vi "Variant to Byte Array.vi"(7 "InStruct":bool=TRUE, 8 "Error In":errorcluster, 10 "Byte Stream In":u8[](array[numeric]), 11 "Variant":variant) -> (0 "Error Out":errorcluster, 2 "Byte Stream Out":u8[](array[numeric]))   [LabVIEW 2020, in "TwinCAT ADS.lvlib" / "PLC.lvlib"]
uses:
  <userlib>/PMA/High Level/PLC/PLC.lvlib
  <vilib>/Utility/error.llb/Error Cluster From Error Code.vi
  <vilib>/ErrorRing/Error Ring.xnode
  <vilib>/Utility/Data Type/NI_Data Type.lvlib
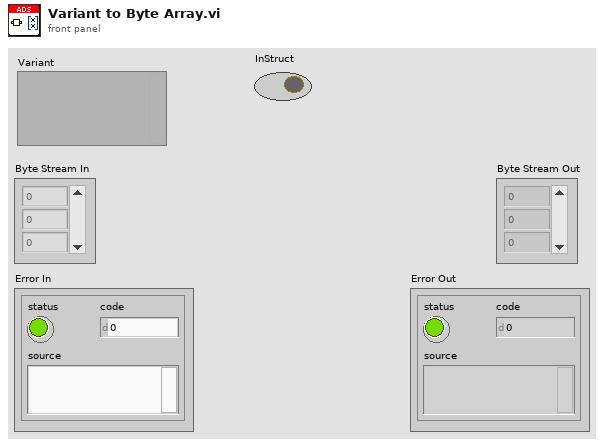
[diagram p1: front panel]
types:
  T1 = typedef "NI_Data Type.lvlib/Data Type.ctl" = enum8{"Invalid Type", "Void", "I8", "I16", "I32", "I64", "U8", "U16", "U32", "U64", "Single Float", "Double Float", "Extended Float", "Single Complex", "Double Complex", "Extended Complex", "Enum U8", "Enum U16", "Enum U32", "Enum U64", "Single Float With Unit", "Double Float With Unit", "Extended Float With Unit", "Single Complex with Unit", "Double Complex with Unit", "Extended Complex with Unit", "Boolean", "String", "Path", "Picture", "Tag", "Array", "Cluster", "Variant", "LV Variant", "Waveform", "Timestamp", "Digital Waveform", "Digital Data", "ExpressData", "Refnum", "External Data", "VI", "Poly VI", "LabVIEW Class Instance", "Fixed Point", "Set Collection", "Map Collection"}
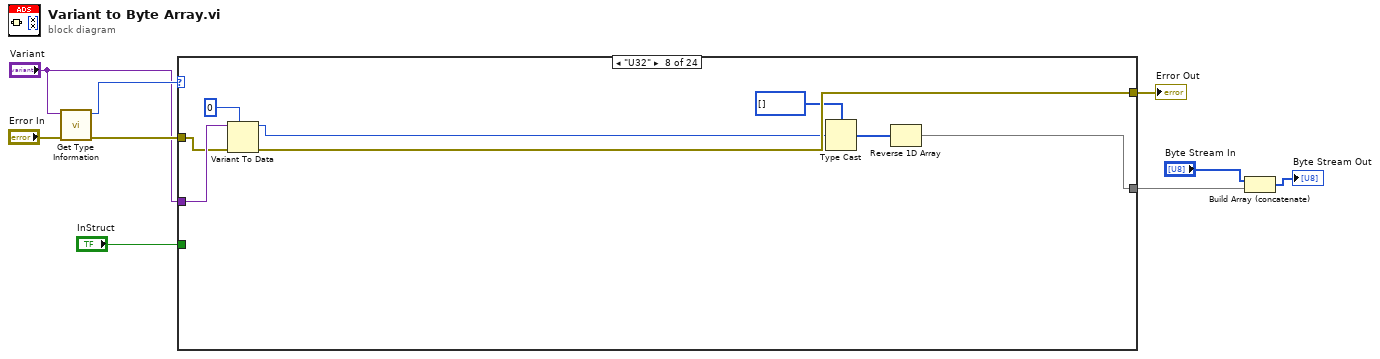
[diagram p0: block diagram]
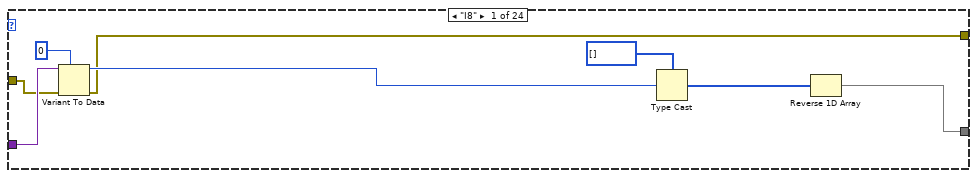
[diagram p2: hidden frame]
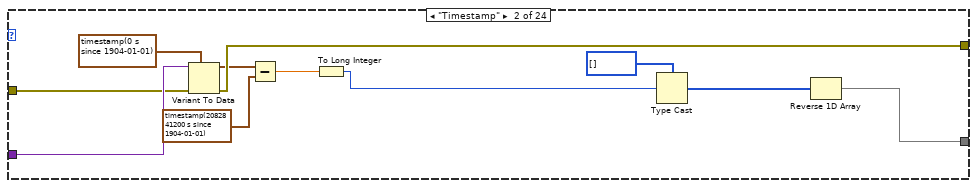
[diagram p3: hidden frame]
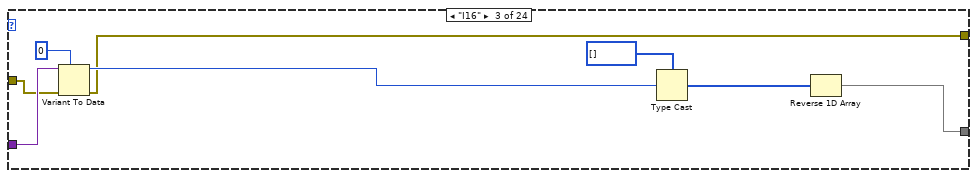
[diagram p4: hidden frame]
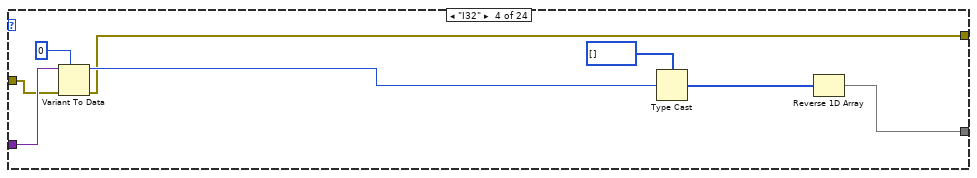
[diagram p5: hidden frame]
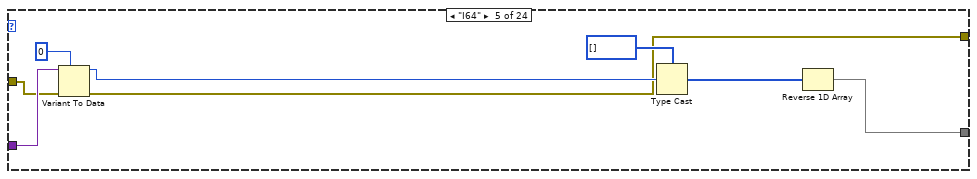
[diagram p6: hidden frame]
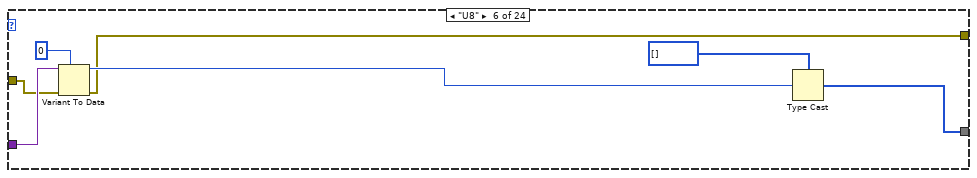
[diagram p7: hidden frame]
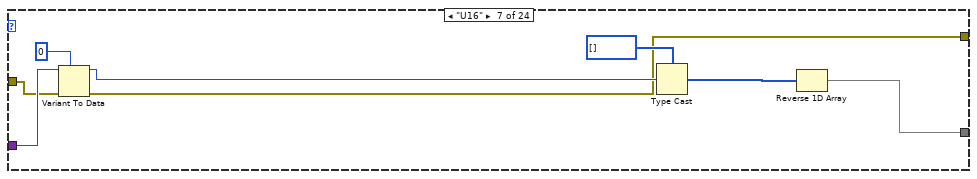
[diagram p8: hidden frame]
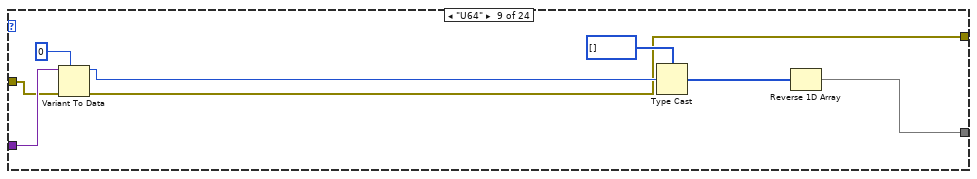
[diagram p9: hidden frame]
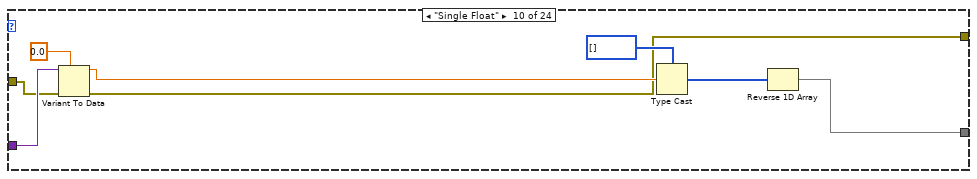
[diagram p10: hidden frame]
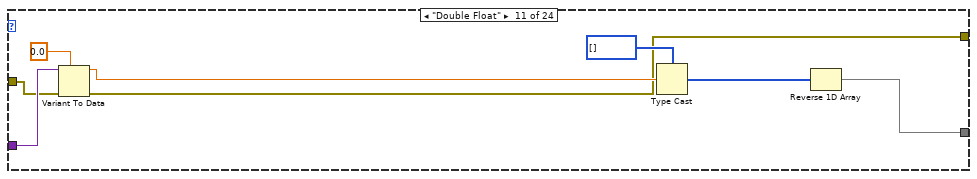
[diagram p11: hidden frame]
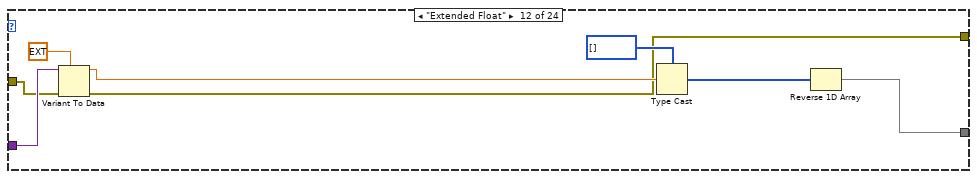
[diagram p12: hidden frame]
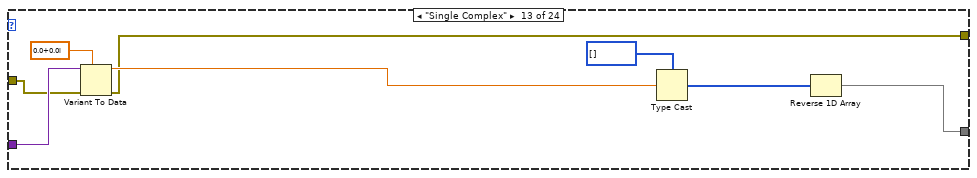
[diagram p13: hidden frame]
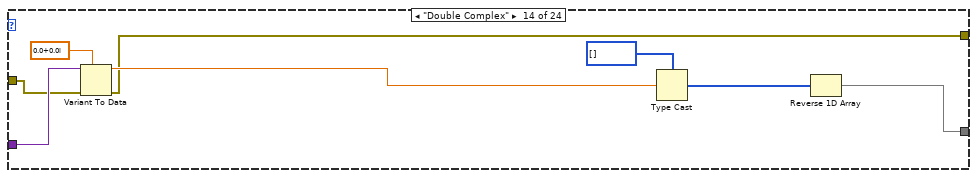
[diagram p14: hidden frame]
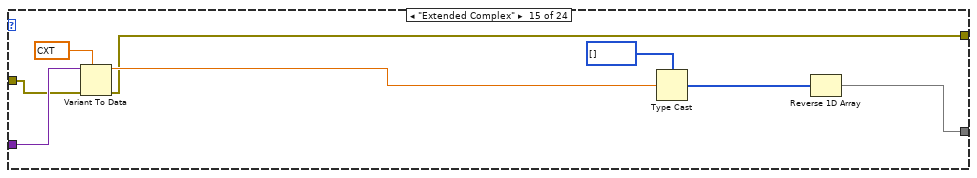
[diagram p15: hidden frame]
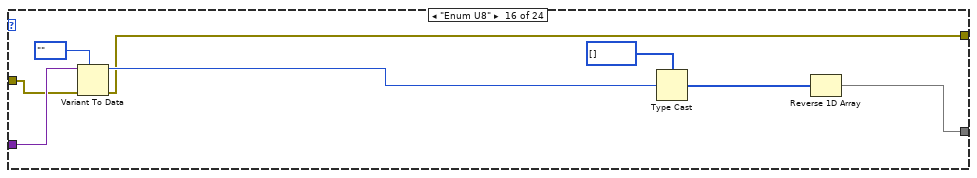
[diagram p16: hidden frame]
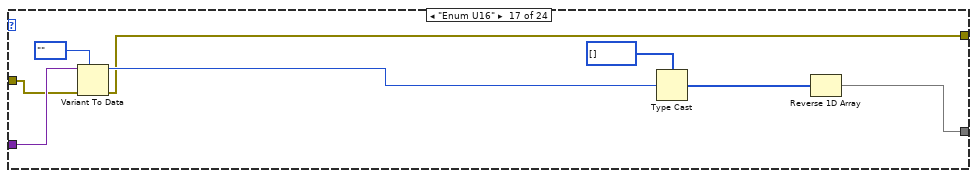
[diagram p17: hidden frame]
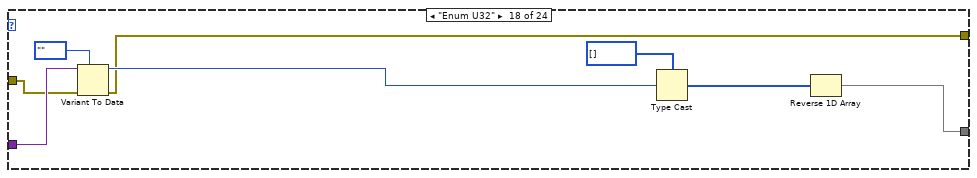
[diagram p18: hidden frame]
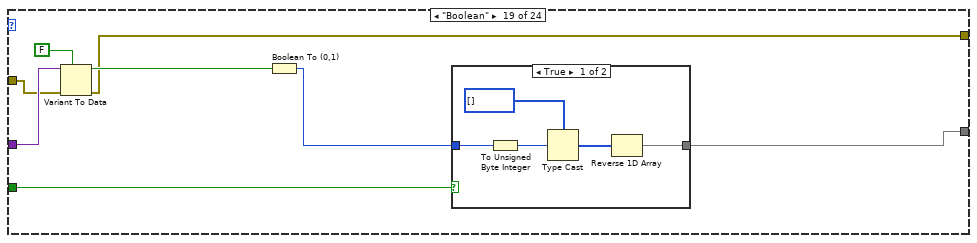
[diagram p19: hidden frame]
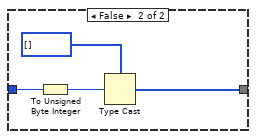
[diagram p20: hidden frame]
diagram:
  n1 = call <vilib>:"Get Type Information.vi"("error in (no error)"="Error In", "variant"="Variant") -> ("error out"=w8:errorcluster, "type"=w9:T1)  [unwired: 5 in, 3 out]
  n2 = case shown="\"U32\"" w9 {
    selector: w9 -> [_ _ _ _ _ _ _ _ _ _ _ _ _ _ _ _ _ _ _ _ _ _ _ w243]
    tunnel: "Variant" -> [w17 w28 w36 w44 w52 w59 w67 w74 w83 w91 w99 w107 w115 w123 w131 w139 w147 w155 w163 w181 w184 w203 _ _]
    tunnel: [w10 w22 w29 w37 w45 w53 w60 w68 w76 w84 w92 w100 w108 w116 w124 w132 w140 w148 w158 w174 w182 w208 _ _] -> w2
    tunnel: w8 -> [w12 w24 w31 w40 w48 w55 w63 w70 w79 w87 w94 w102 w110 w118 w126 w134 w142 w150 w160 w177 w188 w206 w242 _]
    tunnel: [w11 w23 w30 w39 w47 w54 w62 w75 w78 w86 w93 w101 w109 w117 w125 w133 w141 w149 w159 w176 w183 w207 w242 w244] -> w4
    tunnel: "InStruct" -> [_ _ _ _ _ _ _ _ _ _ _ _ _ _ _ _ _ _ w156 _ _ _ _ _]
    frame "I8" {
      n3 = Variant To Data(error in=w12, type=i8 0, Variant=w17) -> (data=w15:i8, error out=w11:errorcluster)
      n4 = Type Cast(type=u8[] [] ("Byte Stream In"), x=w15) -> (*(type *) &x=w13:u8[])
      n5 = Reverse 1D Array(array=w13) -> (reversed array=w10:u8[])
    }
    frame "Timestamp" {
      n6 = Variant To Data(error in=w24, type=timestamp(0 s since 1904-01-01), Variant=w28) -> (data=w21:timestamp, error out=w23:errorcluster)
      n7 = Subtract(x=w21, y=timestamp(2082841200 s since 1904-01-01) ("Time Stamp")) -> (x-y=w19:dbl)
      n8 = To Long Integer(number=w19) -> (32bit integer=w18:i32)
      n9 = Type Cast(type=u8[] [] ("Byte Stream In"), x=w18) -> (*(type *) &x=w25:u8[])
      n10 = Reverse 1D Array(array=w25) -> (reversed array=w22:u8[])
    }
    frame "I16" {
      n11 = Variant To Data(error in=w31, type=i16 0, Variant=w36) -> (data=w34:i16, error out=w30:errorcluster)
      n12 = Type Cast(type=u8[] [] ("Byte Stream In"), x=w34) -> (*(type *) &x=w32:u8[])
      n13 = Reverse 1D Array(array=w32) -> (reversed array=w29:u8[])
    }
    frame "I32" {
      n14 = Variant To Data(error in=w40, type=0, Variant=w44) -> (data=w42:i32, error out=w39:errorcluster)
      n15 = Type Cast(type=u8[] [] ("Byte Stream In"), x=w42) -> (*(type *) &x=w38:u8[])
      n16 = Reverse 1D Array(array=w38) -> (reversed array=w37:u8[])
    }
    frame "I64" {
      n17 = Variant To Data(error in=w48, type=i64 0, Variant=w52) -> (data=w50:i64, error out=w47:errorcluster)
      n18 = Type Cast(type=u8[] [] ("Byte Stream In"), x=w50) -> (*(type *) &x=w46:u8[])
      n19 = Reverse 1D Array(array=w46) -> (reversed array=w45:u8[])
    }
    frame "U8" {
      n20 = Variant To Data(error in=w55, type=u8 0, Variant=w59) -> (data=w57:u8, error out=w54:errorcluster)
      n21 = Type Cast(type=u8[] [] ("Byte Stream In"), x=w57) -> (*(type *) &x=w53:u8[])
    }
    frame "U16" {
      n22 = Variant To Data(error in=w63, type=u16 0, Variant=w67) -> (data=w65:u16, error out=w62:errorcluster)
      n23 = Type Cast(type=u8[] [] ("Byte Stream In"), x=w65) -> (*(type *) &x=w61:u8[])
      n24 = Reverse 1D Array(array=w61) -> (reversed array=w60:u8[])
    }
    frame "U32" {
      n25 = Variant To Data(error in=w70, type=u32 0, Variant=w74) -> (data=w72:u32, error out=w75:errorcluster)
      n26 = Type Cast(type=u8[] [] ("Byte Stream In"), x=w72) -> (*(type *) &x=w69:u8[])
      n27 = Reverse 1D Array(array=w69) -> (reversed array=w68:u8[])
    }
    frame "U64" {
      n28 = Variant To Data(error in=w79, type=u64 0, Variant=w83) -> (data=w81:u64, error out=w78:errorcluster)
      n29 = Type Cast(type=u8[] [] ("Byte Stream In"), x=w81) -> (*(type *) &x=w77:u8[])
      n30 = Reverse 1D Array(array=w77) -> (reversed array=w76:u8[])
    }
    frame "Single Float" {
      n31 = Variant To Data(error in=w87, type=sgl 0.0, Variant=w91) -> (data=w89:sgl, error out=w86:errorcluster)
      n32 = Type Cast(type=u8[] [] ("Byte Stream In"), x=w89) -> (*(type *) &x=w85:u8[])
      n33 = Reverse 1D Array(array=w85) -> (reversed array=w84:u8[])
    }
    frame "Double Float" {
      n34 = Variant To Data(error in=w94, type=0.0, Variant=w99) -> (data=w97:dbl, error out=w93:errorcluster)
      n35 = Type Cast(type=u8[] [] ("Byte Stream In"), x=w97) -> (*(type *) &x=w95:u8[])
      n36 = Reverse 1D Array(array=w95) -> (reversed array=w92:u8[])
    }
    frame "Extended Float" {
      n37 = Variant To Data(error in=w102, type=ext 0.0, Variant=w107) -> (data=w105:ext, error out=w101:errorcluster)
      n38 = Type Cast(type=u8[] [] ("Byte Stream In"), x=w105) -> (*(type *) &x=w103:u8[])
      n39 = Reverse 1D Array(array=w103) -> (reversed array=w100:u8[])
    }
    frame "Single Complex" {
      n40 = Variant To Data(error in=w110, type=csg 0.0+0.0i, Variant=w115) -> (data=w113:csg, error out=w109:errorcluster)
      n41 = Type Cast(type=u8[] [] ("Byte Stream In"), x=w113) -> (*(type *) &x=w111:u8[])
      n42 = Reverse 1D Array(array=w111) -> (reversed array=w108:u8[])
    }
    frame "Double Complex" {
      n43 = Variant To Data(error in=w118, type=cdb 0.0+0.0i, Variant=w123) -> (data=w121:cdb, error out=w117:errorcluster)
      n44 = Type Cast(type=u8[] [] ("Byte Stream In"), x=w121) -> (*(type *) &x=w119:u8[])
      n45 = Reverse 1D Array(array=w119) -> (reversed array=w116:u8[])
    }
    frame "Extended Complex" {
      n46 = Variant To Data(error in=w126, type=cxt 0.0+0.0i, Variant=w131) -> (data=w129:cxt, error out=w125:errorcluster)
      n47 = Type Cast(type=u8[] [] ("Byte Stream In"), x=w129) -> (*(type *) &x=w127:u8[])
      n48 = Reverse 1D Array(array=w127) -> (reversed array=w124:u8[])
    }
    frame "Enum U8" {
      n49 = Variant To Data(error in=w134, type=enum8{""}."", Variant=w139) -> (data=w137:enum8{""}, error out=w133:errorcluster)
      n50 = Type Cast(type=u8[] [] ("Byte Stream In"), x=w137) -> (*(type *) &x=w135:u8[])
      n51 = Reverse 1D Array(array=w135) -> (reversed array=w132:u8[])
    }
    frame "Enum U16" {
      n52 = Variant To Data(error in=w142, type=enum16{""}."", Variant=w147) -> (data=w145:enum16{""}, error out=w141:errorcluster)
      n53 = Type Cast(type=u8[] [] ("Byte Stream In"), x=w145) -> (*(type *) &x=w143:u8[])
      n54 = Reverse 1D Array(array=w143) -> (reversed array=w140:u8[])
    }
    frame "Enum U32" {
      n55 = Variant To Data(error in=w150, type=enum32{""}."", Variant=w155) -> (data=w153:enum32{""}, error out=w149:errorcluster)
      n56 = Type Cast(type=u8[] [] ("Byte Stream In"), x=w153) -> (*(type *) &x=w151:u8[])
      n57 = Reverse 1D Array(array=w151) -> (reversed array=w148:u8[])
    }
    frame "Boolean" {
      n58 = Variant To Data(error in=w160, type=FALSE, Variant=w163) -> (data=w161:bool, error out=w159:errorcluster)
      n59 = Boolean To (0,1)(Boolean=w161) -> (0, 1=w157:i16)
      n60 = case shown="True" w156 {
        tunnel: [w165 w171] -> w158
        tunnel: w157 -> [w166 w170]
        frame True {
          n61 = To Unsigned Byte Integer(number=w166) -> (unsigned 8bit integer=w164:u8)
          n62 = Type Cast(type=u8[] [] ("Byte Stream In"), x=w164) -> (*(type *) &x=w167:u8[])
          n63 = Reverse 1D Array(array=w167) -> (reversed array=w165:u8[])
        }
        frame False {
          n64 = To Unsigned Byte Integer(number=w170) -> (unsigned 8bit integer=w169:u8)
          n65 = Type Cast(type=u8[] [] ("Byte Stream In"), x=w169) -> (*(type *) &x=w171:u8[])
        }
      }
    }
    frame "String" {
      n66 = Variant To Data(error in=w177, type="", Variant=w181) -> (data=w179:string, error out=w176:errorcluster)
      n67 = Type Cast(type=u8[] [] ("Byte Stream In"), x=w179) -> (*(type *) &x=w175:u8[])
      n68 = Reshape Array(w175, 80 ("dimension size")) -> (w174:u8[])
    }
    frame "Cluster" {
      (unwired) u8 0
      n69 = Variant To Flattened String(Variant=w184) -> (data string=w185:string)  [unwired: 1 out]
      n70 = call <vilib>:"Get Cluster Information.vi"("error in (no error)"=w188, "variant"=w184) -> ("error out"=w186:errorcluster, "cluster elements"=w187:variant[])  [unwired: 8 in]
      n71 = for {
        tunnel: w187 -> [w197] mode=indexing
        shift-right: [w201] -> w183
        shift-left: w186 -> [w199]
        tunnel: [w190] -> w189 mode=concatenating
        shift-right: [w196] -> _
        shift-left: w185 -> [w195]
        n72 = Variant To Flattened String(Variant=w197) -> (1:w200:i16[])  [unwired: 1 out]
        n73 = Flattened String To Variant(4:w199, 6:w195, 7:w200) -> (0:w198:errorcluster, 3:w194:variant)
        n74 = Variant To Flattened String(Variant=w194) -> (data string=w193:string)  [unwired: 1 out]
        n75 = call <userlib>:"Variant to Byte Array.vi"("InStruct"=TRUE, "Error In"=w198, "Variant"=w194) -> ("Error Out"=w201:errorcluster, "Byte Stream Out"=w190:u8[])  [unwired: 7 in]
        n76 = String Length(string=w193) -> (length=w192:i32)
        n77 = String Subset(string=w195, offset (0)=w192) -> (substring=w196:string)  [unwired: 1 in]
      }
      n78 = Build Array (concatenate)(w189) -> (w182:u8[])
    }
    frame "Array" {
      n79 = call <vilib>:"Get Array Information.vi"("error in (no error)"=w206, "variant"=w203) -> ("error out"=w205:errorcluster, "number of dimensions"=w204:i32)  [unwired: 6 in, 2 out]
      n80 = case shown="1" w204 {
        tunnel: [u8[] [] ("Byte Stream Out") w218 w231] -> w208
        tunnel: [w210 w217 w230] -> w207
        tunnel: w205 -> [w210 w213 w227]
        tunnel: w203 -> [_ w214 w228]
        tunnel: TRUE ("InStruct") -> [_ w211 w224]
        frame 0, Default {
        }
        frame 1 {
          n81 = Variant To Data(error in=w213, type=variant[] [], Variant=w214) -> (data=w216:variant[], error out=w212:errorcluster)
          n82 = for {
            shift-right: [w222] -> w217
            shift-left: w212 -> [w220]
            tunnel: [w223] -> w218 mode=concatenating
            tunnel: w216 -> [w221] mode=indexing
            tunnel: w211 -> [w219]
            n83 = call <userlib>:"Variant to Byte Array.vi"("InStruct"=w219, "Error In"=w220, "Variant"=w221) -> ("Error Out"=w222:errorcluster, "Byte Stream Out"=w223:u8[])  [unwired: 7 in]
          }
        }
        frame 2 {
          n84 = Variant To Data(error in=w227, type=variant[][] [], Variant=w228) -> (data=w225:variant[][], error out=w226:errorcluster)
          n85 = for {
            shift-right: [w235] -> w230
            shift-left: w226 -> [w233]
            tunnel: [w236] -> w231 mode=concatenating
            tunnel: w225 -> [w234] mode=indexing
            tunnel: w224 -> [w232]
            n86 = for {
              tunnel: [w241] -> w236 mode=concatenating
              tunnel: w234 -> [w239] mode=indexing
              shift-right: [w240] -> w235
              shift-left: w233 -> [w238]
              tunnel: w232 -> [w237]
              n87 = call <userlib>:"Variant to Byte Array.vi"("InStruct"=w237, "Error In"=w238, "Variant"=w239) -> ("Error Out"=w240:errorcluster, "Byte Stream Out"=w241:u8[])  [unwired: 7 in]
            }
          }
        }
      }
    }
    frame "Void", "Variant" {
    }
    frame Default {
      n88 = xnode "Error Ring"("parameter 0"=w243) -> ("error out"=w244:errorcluster)
    }
  }
  "Error Out" <- w4
  n89 = Build Array (concatenate)("Byte Stream In", w2) -> (→"Byte Stream Out":u8[])
